vi "6733_write_waveform.vi"(8 "Error In":errorcluster, 9 "Control Task In":refnum<k21>, 10 "Waveform Task In":refnum<k21>, 11 "Inputs":T1 {"Waveform Parameters"."Degree (polynomial only)" min=1}) -> (0 "error out":errorcluster, 2 "counter task out":refnum<k21>, 3 "waveform task out":refnum<k21>)   [LabVIEW 2013]
uses:
  Control 1.ctl
  <vilib>/DAQmx/write.llb/DAQmx Write (Analog 1D DBL NChan 1Samp).vi
  <vilib>/DAQmx/write.llb/DAQmx Write (Analog 1D Wfm NChan NSamp).vi
  <vilib>/DAQmx/create/channels.llb/DAQmx Create Channel (AO-Voltage-Basic).vi
  <vilib>/DAQmx/miscellaneous.llb/DAQmx Fill In Error Info.vi
  <vilib>/Waveform/WDTOps.llb/WDT Append Waveforms DBL.vi
  <vilib>/DAQmx/configure/timing.llb/DAQmx Timing (Sample Clock).vi
  <vilib>/DAQmx/create/channels.llb/DAQmx Create Channel (CO-Pulse Generation-Frequency).vi
  <vilib>/DAQmx/configure/timing.llb/DAQmx Timing (Implicit).vi
  <vilib>/DAQmx/configure/trigger.llb/DAQmx Start Trigger (Digital Edge).vi
  <vilib>/Waveform/WDTOps.llb/WDT Scale Delta t DBL.vi
  <resource>/objmgr/daqmx.rc
panel:
  out "Total Time":dbl
  out "Sample Rate":dbl
  out "element":waveform(dbl)(graph)
  in  "index":i32
  out "Waveforms":waveform(dbl)[](array[waveform])
  out "Max Sample Rate":dbl=1000000.0
  out "# Inactive Channels":i32
  out "# Active Channels":i16
  out "Inactive Channels":tag[](array[tag])
  out "Active Channels":tag[](array[tag])
  out "Samples Written":dbl
  out "Voltage Maximum":dbl
  out "Voltage Minimum":dbl
  out "AO.PhysicalChans":tag[](array[tag])
  out "Active Device":tag
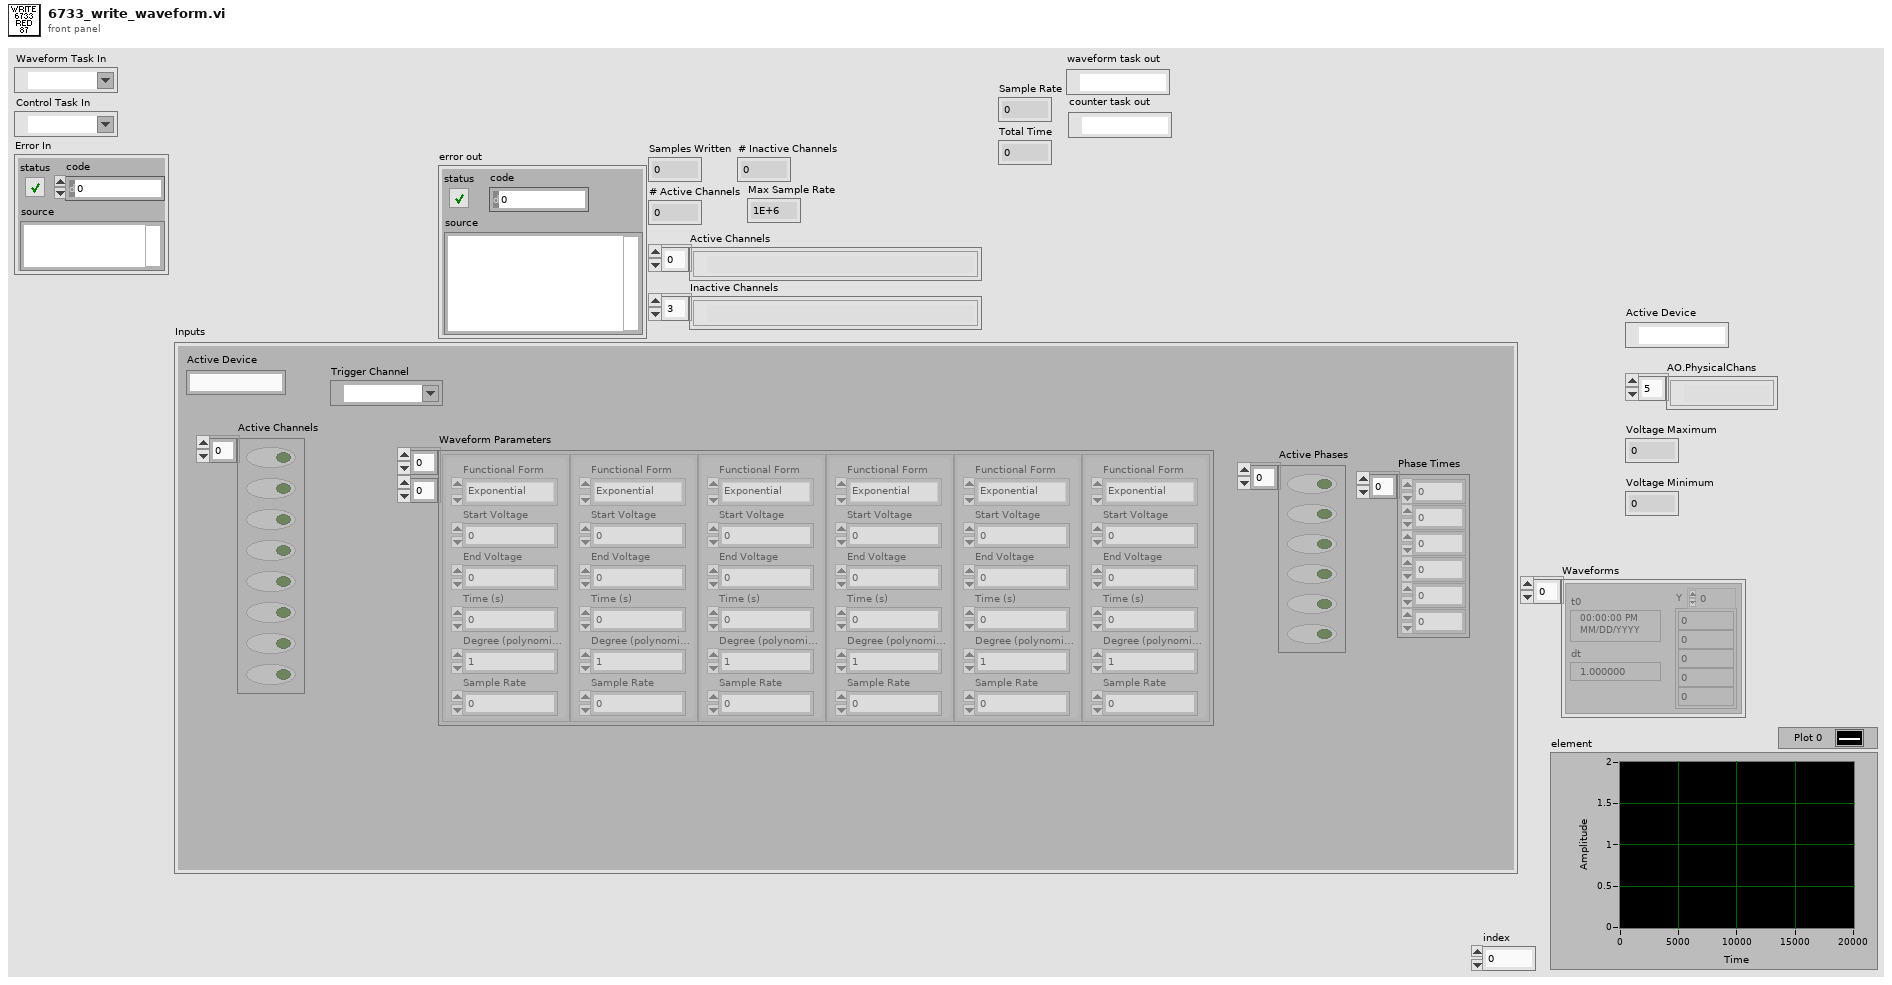
[diagram p1: front panel]
types:
  T1 = cluster{"Active Device":string, "Active Channels":bool[], "Waveform Parameters":cluster{"Functional Form":enum16{"Polynomial", "Exponential"}, "Start Voltage":dbl, "End Voltage":dbl, "Time (s)":dbl, "Degree (polynomial only)":i8, "Sample Rate":dbl}[][], "Active Phases":bool[], "Phase Times":dbl[], "Trigger Channel":tag}
  T2 = typedef "Control 1.ctl" = enum16{"Initialize", "Get Device Information", "Get Active/Inactive Channels", "Maximize Samples / Channel", "Write Waveforms", "Check for Problems", "Clear Old Tasks", "Write to cards"}
  T3 = cluster{"Functional Form":enum16{"Polynomial", "Exponential"}, "Start Voltage":dbl, "End Voltage":dbl, "Time (s)":dbl, "Degree (polynomial only)":i8, "Sample Rate":dbl}[][]
  T4 = cluster{"Functional Form":enum16{"Polynomial", "Exponential"}, "Start Voltage":dbl, "End Voltage":dbl, "Time (s)":dbl, "Degree (polynomial only)":i8, "Sample Rate":dbl}[]
  T5 = cluster{"Functional Form":enum16{"Polynomial", "Exponential"}, "Start Voltage":dbl, "End Voltage":dbl, "Time (s)":dbl, "Degree (polynomial only)":i8, "Sample Rate":dbl}
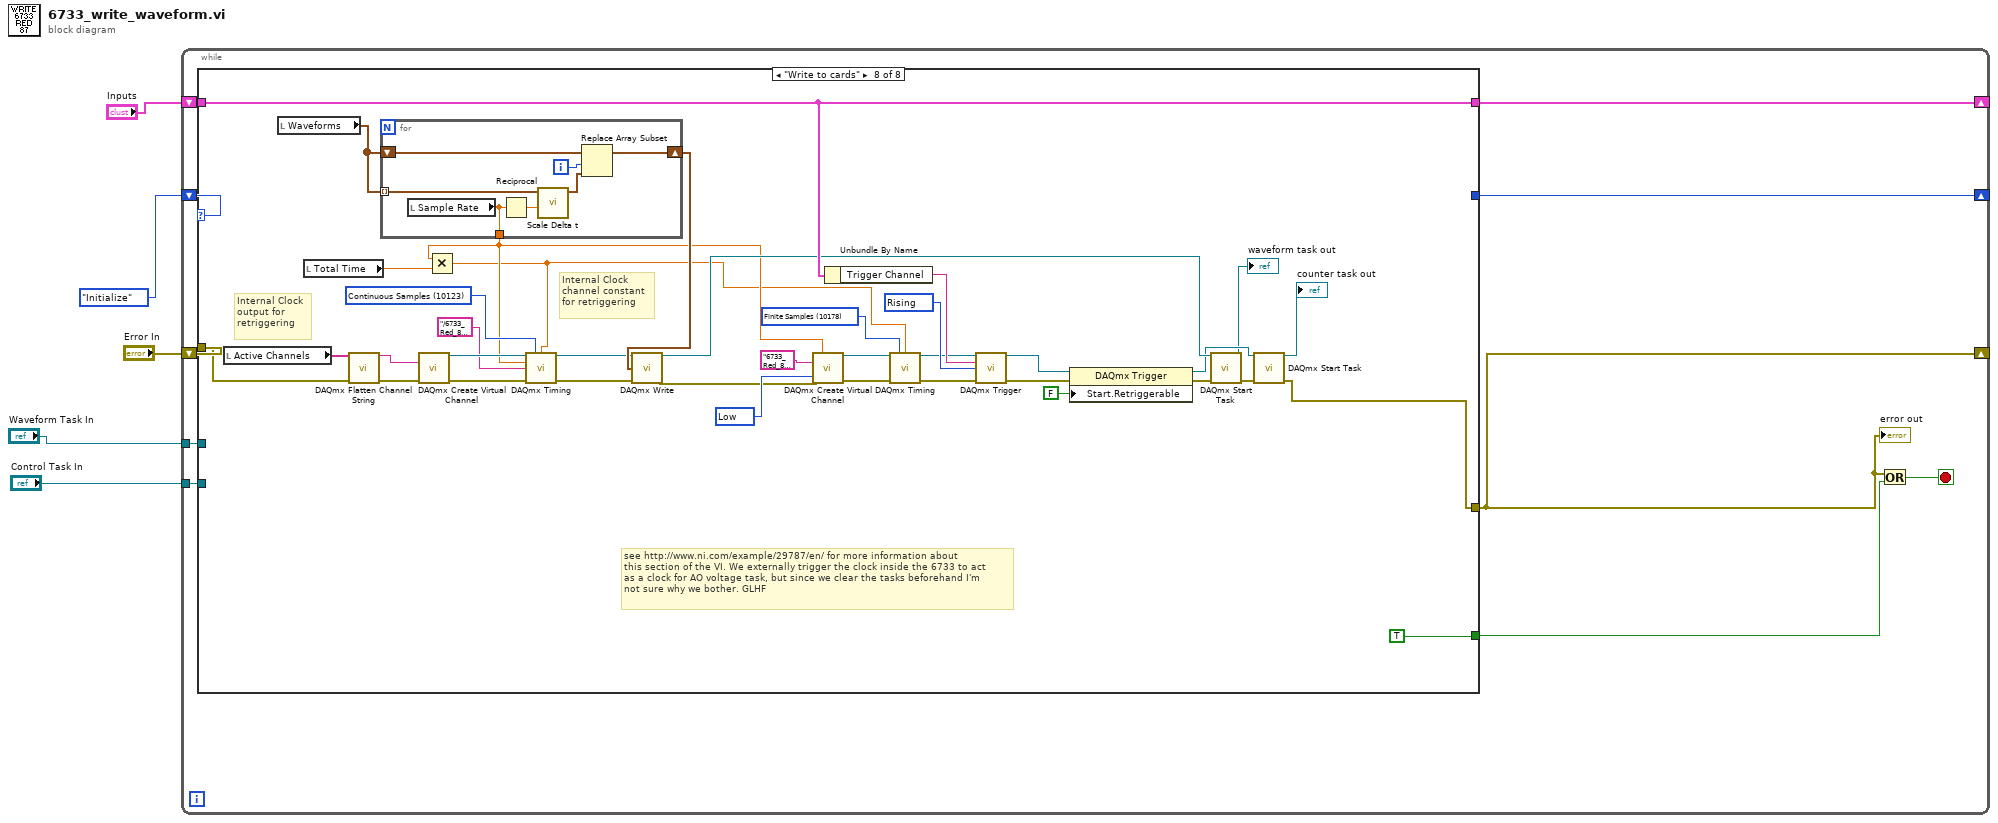
[diagram p0: block diagram]
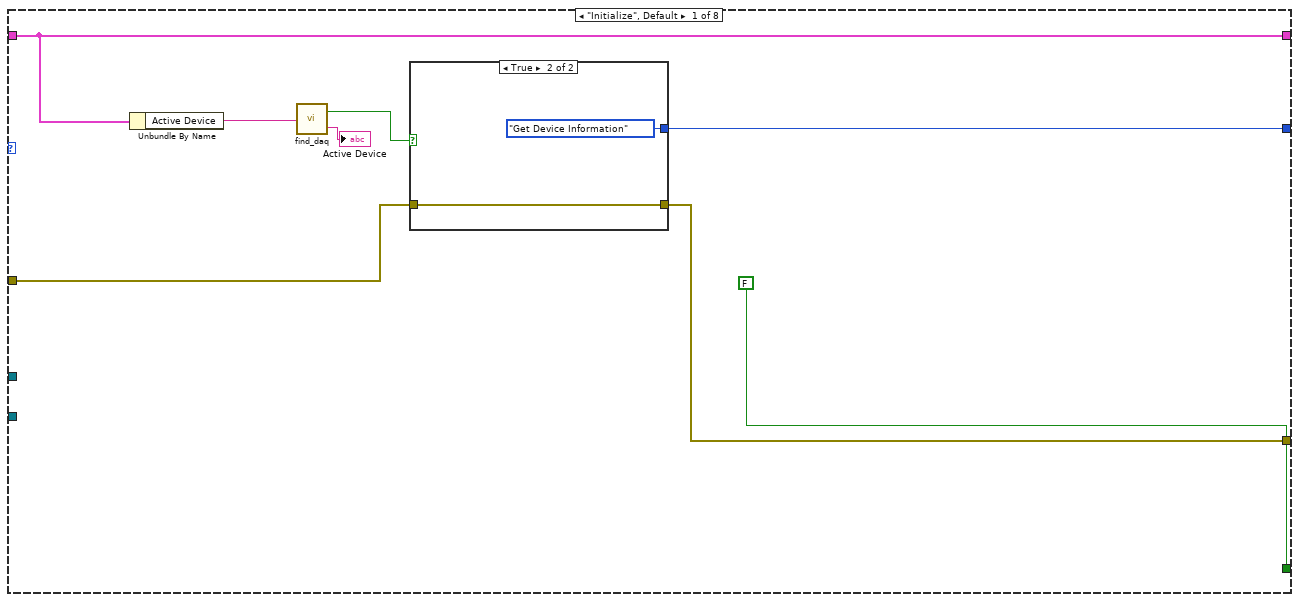
[diagram p2: hidden frame]
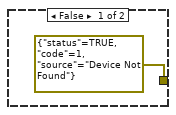
[diagram p3: hidden frame]
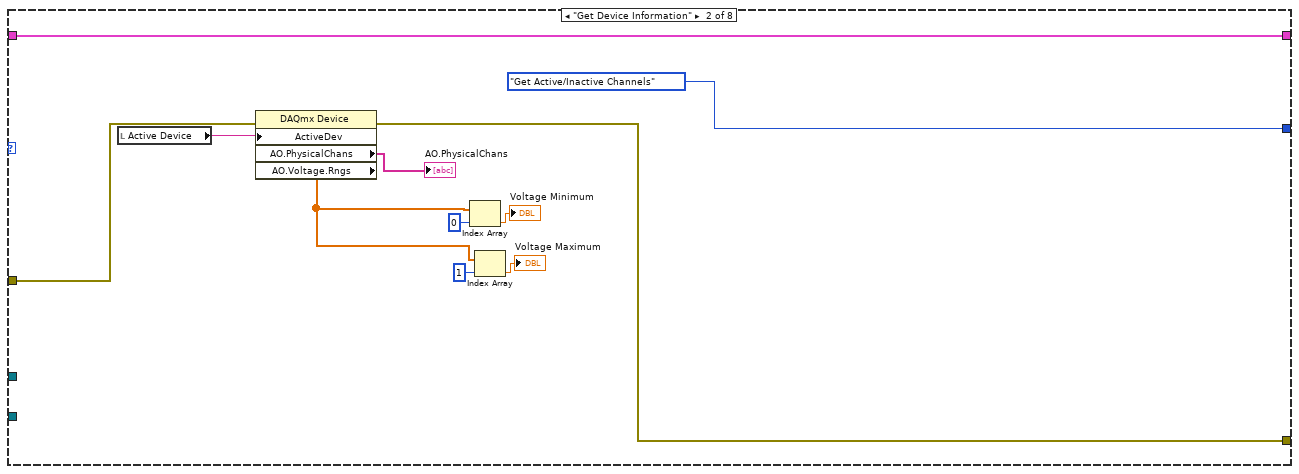
[diagram p4: hidden frame]
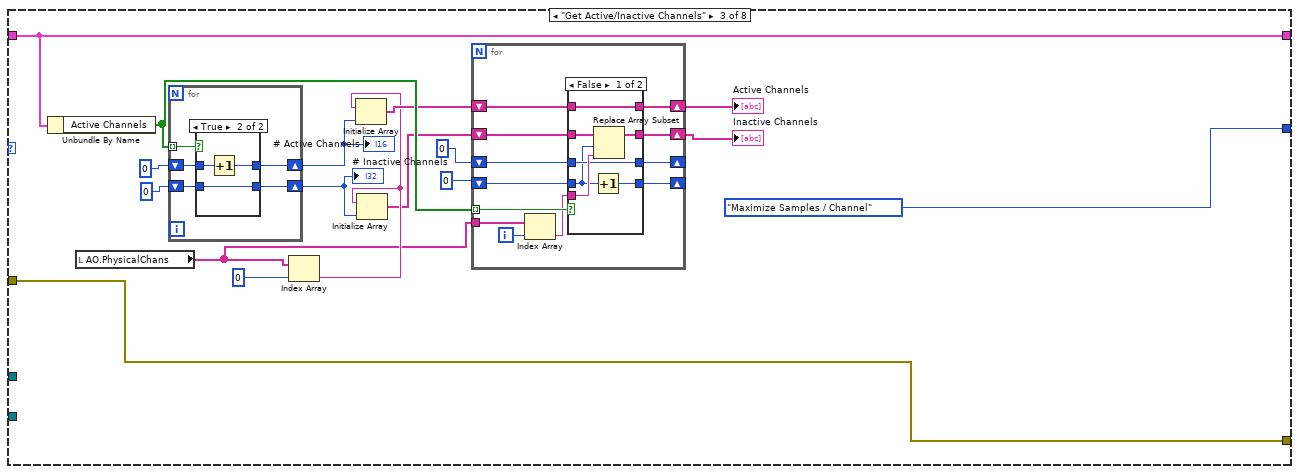
[diagram p5: hidden frame]
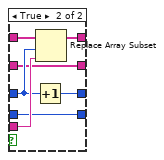
[diagram p6: hidden frame]
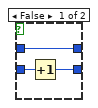
[diagram p7: hidden frame]
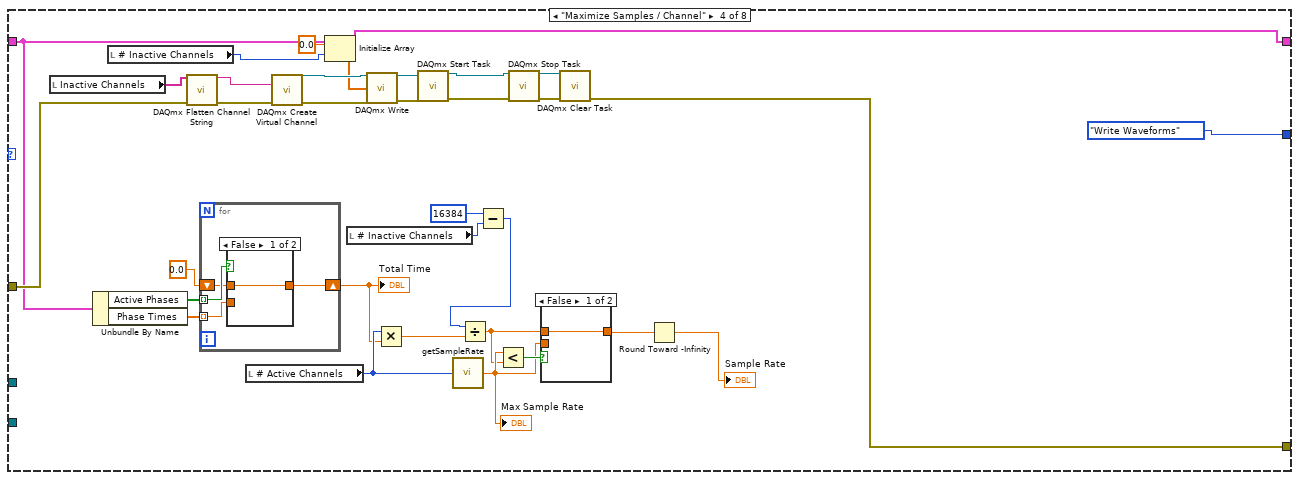
[diagram p8: hidden frame]
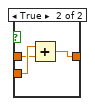
[diagram p10: hidden frame]
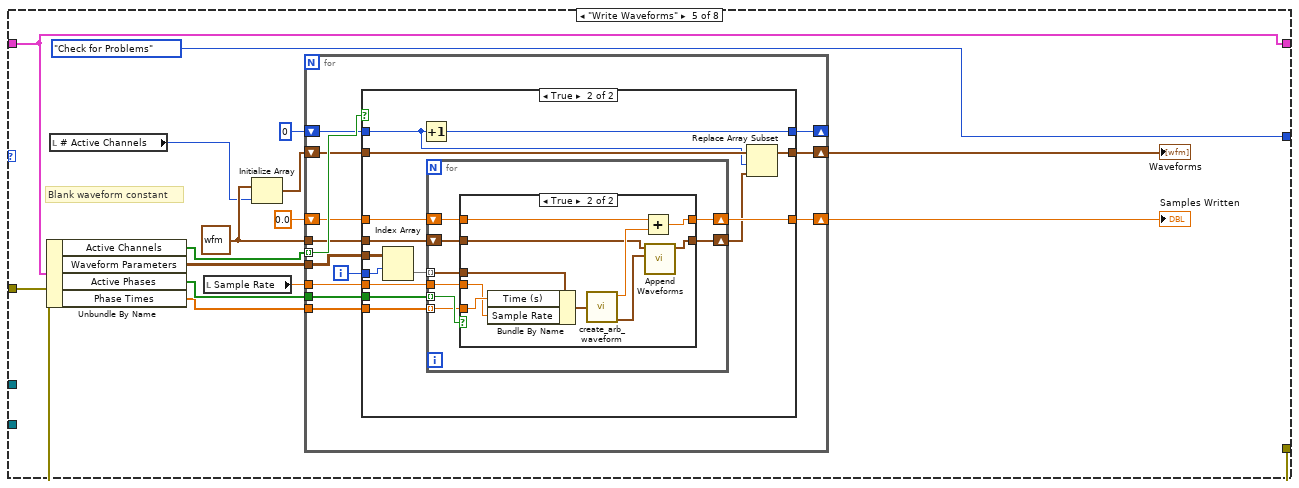
[diagram p11: hidden frame]
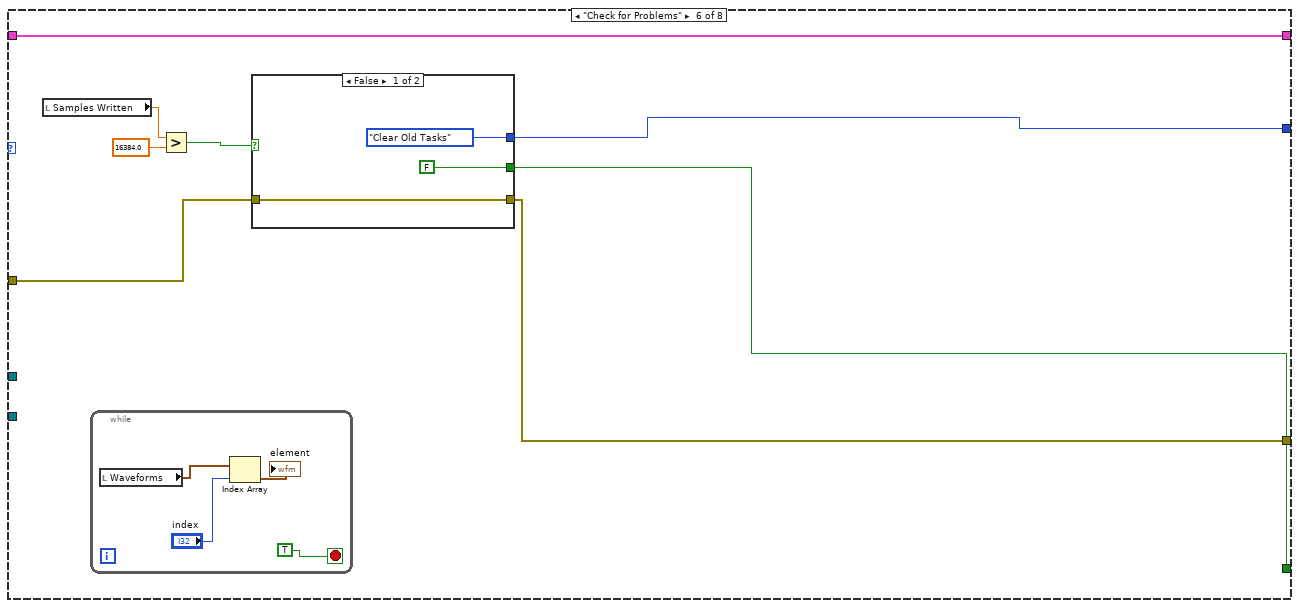
[diagram p14: hidden frame]
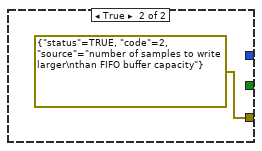
[diagram p15: hidden frame]
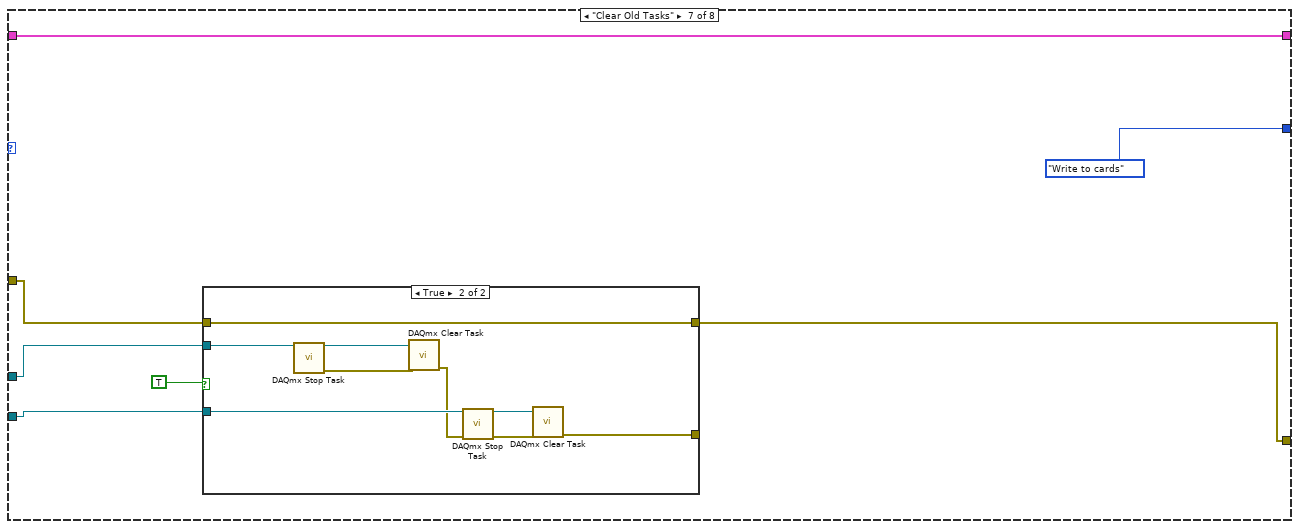
[diagram p16: hidden frame]
diagram:
  n1 = while {
    shift-right: [w11] -> _
    shift-left: "Error In" -> [w13]
    shift-right: [w12] -> _
    shift-left: Control_1."Initialize" -> [w15]
    shift-right: [w9] -> _
    shift-left: "Inputs" -> [w14]
    tunnel: "Control Task In" -> [w6]
    tunnel: "Waveform Task In" -> [w7]
    stop <- w10 stop-if-true
    n2 = case shown="\"Write to cards\"" w15 {
      tunnel: w14 -> [w17 w37 w41 w106 w144 w201 w215 w266]
      tunnel: [w20 w28 w52 w110 w147 w202 w218 w237] -> w11
      tunnel: w13 -> [w19 w36 w52 w121 w147 w203 w217 w265]
      tunnel: [w18 Control_1."Get Active/Inactive Channels" Control_1."Maximize Samples / Channel" Control_1."Write Waveforms" Control_1."Check for Problems" w200 Control_1."Write to cards" _] -> w12
      tunnel: [w17 w37 w41 w106 w144 w201 w215 w266] -> w9
      tunnel: [FALSE ("y") _ _ _ _ w199 _ TRUE ("y")] -> w8
      tunnel: w7 -> [_ _ _ _ _ _ w221 _]
      tunnel: w6 -> [_ _ _ _ _ _ w219 _]
      frame "Initialize", Default {
        n3 = Unbundle By Name(w17) -> ("Active Device"=w23:string)
        n4 = call "find_daq.vi"("Device Name"=w23) -> ("Device Present"=w21:bool, "DAQmx Device Name"=→"Active Device":tag)
        n5 = case shown="True" w21 {
          tunnel: [errorcluster {"status"=TRUE, "code"=1, "source"="Device Not Found"} ("error in (no error)") w26] -> w20
          tunnel: w19 -> [_ w26]
          tunnel: [_ Control_1."Get Device Information"] -> w18
          frame False {
          }
          frame True {
          }
        }
      }
      frame "Get Device Information" {
        n6 = local read "Active Device"() -> (w35:tag)
        n7 = property class="DAQmx Device"(error in=w36, "ActiveDev"=w35) -> (error out=w28:errorcluster, "AO.PhysicalChans"=→"AO.PhysicalChans":tag[], "AO.Voltage.Rngs"=w30:dbl[])  [unwired: 1 in, 1 out]
        n8 = Index Array(array=w30, index=0) -> (element=→"Voltage Minimum":dbl)
        n9 = Index Array(array=w30, index=1) -> (element=→"Voltage Maximum":dbl)
      }
      frame "Get Active/Inactive Channels" {
        n10 = Unbundle By Name(w41) -> ("Active Channels"=w51:bool[])
        n11 = local read "AO.PhysicalChans"() -> (w45:tag[])
        n12 = for {
          shift-right: [w85] -> w50
          shift-left: i16 0 -> [w84]
          shift-right: [w83] -> w49
          shift-left: 0 -> [w82]
          tunnel: w51 -> [w81] mode=indexing
          n13 = case shown="True" w81 {
            tunnel: [w86 w91] -> w85
            tunnel: w84 -> [w86 w90]
            tunnel: [w88 w89] -> w83
            tunnel: w82 -> [w87 w89]
            frame False {
              n14 = Increment(x=w87) -> (x+1=w88:i32)
            }
            frame True {
              n15 = Increment(x=w90) -> (x+1=w91:i16)
            }
          }
        }
        "# Active Channels" <- w50
        "# Inactive Channels" <- w49
        n16 = Index Array(array=w45, index=0) -> (element=w46:tag)
        n17 = Initialize Array(w46, w50) -> (w48:tag[])
        n18 = Initialize Array(w46, w49) -> (w44:tag[])
        n19 = for {
          tunnel: w51 -> [w66] mode=indexing
          shift-right: [w63] -> w40
          shift-left: w48 -> [w64]
          tunnel: w45 -> [w61]
          shift-right: [w59] -> w39
          shift-left: w44 -> [w60]
          shift-right: [w57] -> _
          shift-left: 0 ("index") -> [w58]
          shift-right: [w55] -> _
          shift-left: 0 ("index") -> [w56]
          i -> [w65]
          n20 = Index Array(array=w61, index=w65) -> (element=w62:tag)
          n21 = case shown="False" w66 {
            tunnel: w64 -> [w67 w80]
            tunnel: [w67 w79] -> w63
            tunnel: w62 -> [w73 w78]
            tunnel: w60 -> [w72 w74]
            tunnel: [w71 w74] -> w59
            tunnel: w58 -> [w70 w77]
            tunnel: [w70 w76] -> w57
            tunnel: w56 -> [w69 w75]
            tunnel: [w68 w75] -> w55
            frame False {
              n22 = Increment(x=w69) -> (x+1=w68:i32)
              n23 = Replace Array Subset(array=w72, new element=w73, index=w69) -> (w71:tag[])
            }
            frame True {
              n24 = Increment(x=w77) -> (x+1=w76:i32)
              n25 = Replace Array Subset(array=w80, new element=w78, index=w77) -> (w79:tag[])
            }
          }
        }
        "Active Channels" <- w40
        "Inactive Channels" <- w39
      }
      frame "Maximize Samples / Channel" {
        n26 = local read "Inactive Channels"() -> (w122:tag[])
        n27 = Unbundle By Name(w106) -> ("Active Phases"=w105:bool[], "Phase Times"=w104:dbl[])
        n28 = local read "# Inactive Channels"() -> (w115:i32)
        n29 = call <vilib>:"DAQmx Flatten Channel String.vi"("names in"=w122, "error in"=w121) -> ("names out"=w120:string, "error out"=w123:errorcluster)  [unwired: 12 in]
        n30 = for {
          tunnel: w105 -> [w129] mode=indexing
          tunnel: w104 -> [w128] mode=indexing
          shift-right: [w126] -> w97
          shift-left: 0.0 -> [w127]
          n31 = case shown="False" w129 {
            tunnel: w128 -> [_ w133]
            tunnel: w127 -> [w130 w132]
            tunnel: [w130 w131] -> w126
            frame False {
            }
            frame True {
              n32 = Add(x=w133, y=w132) -> (x+y=w131:dbl)
            }
          }
        }
        "Total Time" <- w97
        n33 = local read "# Active Channels"() -> (w98:i16)
        n34 = call-poly <vilib>:"DAQmx Create Virtual Channel.vi"("physical channels"=w120, "error in"=w123) -> ("task out"=w119:refnum<k21>, "error out"=w118:errorcluster)  [unwired: 12 in]
        n35 = Initialize Array(0.0 ("element"), w115) -> (w113:dbl[])
        n36 = local read "# Inactive Channels"() -> (w93:i32)
        n37 = call-poly <vilib>:"DAQmx Write.vi"("task/channels in"=w119, "data"=w113, "error in"=w118) -> ("task out"=w116:refnum<k21>, "error out"=w117:errorcluster)  [unwired: 10 in, 1 out]
        n38 = Multiply(x=w98, y=w97) -> (x*y=w99:dbl)
        n39 = call <vilib>:"DAQmx Start Task.vi"("task/channels in"=w116, "error in"=w117) -> ("task out"=w108:refnum<k21>, "error out"=w109:errorcluster)  [unwired: 12 in]
        n40 = call "getSampleRate.vi"("Number of active channels"=w98) -> ("Sample Rate"=w101:dbl)
        "Max Sample Rate" <- w101
        n41 = Subtract(x=16384, y=w93) -> (x-y=w92:i32)
        n42 = Divide(x=w92, y=w99) -> (x/y=w100:dbl)
        n43 = Less?(x=w101, y=w100) -> (x < y?=w102:bool)
        n44 = call <vilib>:"DAQmx Stop Task.vi"("task/channels in"=w108, "error in"=w109) -> ("task out"=w112:refnum<k21>, "error out"=w111:errorcluster)  [unwired: 12 in]
        n45 = case shown="False" w102 {
          tunnel: [w124 w125] -> w95
          tunnel: w101 -> [_ w125]
          tunnel: w100 -> [w124 _]
          frame False {
          }
          frame True {
          }
        }
        n46 = call <vilib>:"DAQmx Clear Task.vi"("task in"=w112, "error in"=w111) -> ("error out"=w110:errorcluster)  [unwired: 13 in]
        n47 = Round Toward -Infinity(1:w95) -> (0:→"Sample Rate":dbl)
      }
      frame "Write Waveforms" {
        w141 = waveform(dbl) {"t0"=timestamp(0 s since 1904-01-01), "dt"=1.0, "Y"=[]}
        # "Blank waveform constant"
        n48 = Unbundle By Name(w144) -> ("Active Channels"=w136:bool[], "Waveform Parameters"=w148:T3, "Active Phases"=w142:bool[], "Phase Times"=w137:dbl[])
        n49 = local read "# Active Channels"() -> (w134:i16)
        n50 = local read "Sample Rate"() -> (w135:dbl)
        n51 = Initialize Array(w141, w134) -> (w139:waveform(dbl)[])
        n52 = for {
          tunnel: w136 -> [w161] mode=indexing
          tunnel: w148 -> [w159]
          shift-right: [w158] -> w146
          shift-left: 0.0 -> [w157]
          tunnel: w142 -> [w156]
          tunnel: w141 -> [w155]
          shift-right: [w153] -> _
          shift-left: 0 -> [w154]
          shift-right: [w151] -> w138
          shift-left: w139 -> [w152]
          tunnel: w137 -> [w150]
          tunnel: w135 -> [w149]
          i -> [w160]
          n53 = case shown="True" w161 {
            tunnel: w160 -> [_ w178]
            tunnel: w159 -> [_ w177]
            tunnel: [w164 w176] -> w158
            tunnel: w157 -> [w164 w175]
            tunnel: w156 -> [_ w173]
            tunnel: w155 -> [_ w172]
            tunnel: w154 -> [w163 w169]
            tunnel: [w163 w171] -> w153
            tunnel: w152 -> [w162 w170]
            tunnel: [w162 w167] -> w151
            tunnel: w150 -> [_ w166]
            tunnel: w149 -> [_ w165]
            frame False {
            }
            frame True {
              n54 = Index Array(array=w177, index (row)=w178) -> (element=w174:T4)  [unwired: 1 in]
              n55 = Increment(x=w169) -> (x+1=w171:i32)
              n56 = for {
                shift-right: [w186] -> w176
                shift-left: w175 -> [w185]
                tunnel: w174 -> [w184] mode=indexing
                shift-right: [w182] -> w168
                shift-left: w172 -> [w183]
                tunnel: w173 -> [w181] mode=indexing
                tunnel: w166 -> [w180] mode=indexing
                tunnel: w165 -> [w179]
                n57 = case shown="True" w181 {
                  tunnel: [w188 w197] -> w186
                  tunnel: w185 -> [w188 w196]
                  tunnel: w184 -> [_ w192]
                  tunnel: w183 -> [w187 w194]
                  tunnel: [w187 w193] -> w182
                  tunnel: w180 -> [_ w191]
                  tunnel: w179 -> [_ w189]
                  frame False {
                  }
                  frame True {
                    n58 = Bundle By Name(cluster=w192, "Time (s)"=w191, "Sample Rate"=w189) -> (w190:T5)
                    n59 = call "create_arb_waveform.vi"("Waveform Parameters"=w190) -> ("Samples to Write"=w198:dbl, "output waveform"=w195:waveform(dbl))  [unwired: 2 out]
                    n60 = Add(x=w196, y=w198) -> (x+y=w197:dbl)
                    n61 = call-poly <vilib>:"Append Waveforms.vi"("waveform B"=w195, "waveform A"=w194) -> ("waveform out"=w193:waveform(dbl))  [unwired: 8 in, 1 out]
                  }
                }
              }
              n62 = Replace Array Subset(array=w170, new element=w168, index=w169) -> (w167:waveform(dbl)[])
            }
          }
        }
        "Samples Written" <- w146
        "Waveforms" <- w138
      }
      frame "Check for Problems" {
        n63 = local read "Samples Written"() -> (w206:dbl)
        n64 = while {
          stop <- TRUE stop-if-true
          n65 = local read "Waveforms"() -> (w210:waveform(dbl)[])
          n66 = Index Array(array=w210, index="index") -> (element=→"element":waveform(dbl))
        }
        n67 = Greater?(x=w206, y=16384.0) -> (0:w205:bool)
        n68 = case shown="False" w205 {
          tunnel: w203 -> [w213 _]
          tunnel: [w213 errorcluster {"status"=TRUE, "code"=2, "source"="number of samples to write larger\nthan FIFO buffer capacity"} ("error in (no error)")] -> w202
          tunnel: [Control_1."Clear Old Tasks" _] -> w200
          tunnel: [FALSE ("y") _] -> w199
          frame False {
          }
          frame True {
          }
        }
      }
      frame "Clear Old Tasks" {
        n69 = case shown="True" TRUE {
          tunnel: w221 -> [_ w231]
          tunnel: w219 -> [_ w229]
          tunnel: [w222 w227] -> w218
          tunnel: w217 -> [w222 w227]
          tunnel: [_ w223] -> _
          frame False {
          }
          frame True {
            n70 = call <vilib>:"DAQmx Stop Task.vi"("task/channels in"=w231) -> ("task out"=w230:refnum<k21>, "error out"=w226:errorcluster)  [unwired: 13 in]
            n71 = call <vilib>:"DAQmx Clear Task.vi"("task in"=w230, "error in"=w226) -> ("error out"=w225:errorcluster)  [unwired: 13 in]
            n72 = call <vilib>:"DAQmx Stop Task.vi"("task/channels in"=w229, "error in"=w225) -> ("task out"=w228:refnum<k21>, "error out"=w224:errorcluster)  [unwired: 12 in]
            n73 = call <vilib>:"DAQmx Clear Task.vi"("task in"=w228, "error in"=w224) -> ("error out"=w223:errorcluster)  [unwired: 13 in]
          }
        }
      }
      frame "Write to cards" {
        w250 = 10280 items=["Rising"=10280, "Falling"=10171] ("edge")
        w257 = 10123 items=["Finite Samples"=10178, "Continuous Samples"=10123, "Hardware Timed Single Point"=12522] ("sample mode")
        w259 = 10178 items=["Finite Samples"=10178, "Continuous Samples"=10123, "Hardware Timed Single Point"=12522] ("sample mode")
        w262 = 10214 items=["High"=10192, "Low"=10214] ("idle state")
        # "see http://www.ni.com/example/29787/en/ for more information about\nthis section of the VI. We externally trigger the clock inside the 6733 to act\nas a clock for AO voltage task, but since we clear the tasks beforehand I'm\nnot sure why we bother. GLHF"
        # "Internal Clock\noutput for\nretriggering"
        # "Internal Clock\nchannel constant\nfor retriggering"
        n74 = local read "Active Channels"() -> (w264:tag[])
        n75 = local read "Waveforms"() -> (w267:waveform(dbl)[])
        n76 = local read "Total Time"() -> (w258:dbl)
        n77 = call <vilib>:"DAQmx Flatten Channel String.vi"("names in"=w264, "error in"=w265) -> ("names out"=w263:string, "error out"=w234:errorcluster)  [unwired: 12 in]
        n78 = for {
          tunnel: w267 -> [w275] mode=indexing
          shift-right: [w269] -> w253
          shift-left: w267 -> [w271]
          tunnel: [w270] -> w240
          i -> [w273]
          n79 = local read "Sample Rate"() -> (w270:dbl)
          n80 = Reciprocal(x=w270) -> (1/x=w274:dbl)
          n81 = call-poly <vilib>:"Scale Delta t.vi"("scale factor"=w274, "waveform in"=w275) -> ("waveform out"=w272:waveform(dbl))  [unwired: 8 in, 1 out]
          n82 = Replace Array Subset(array=w271, new element=w272, index=w273) -> (w269:waveform(dbl)[])
        }
        n83 = call-poly <vilib>:"DAQmx Create Virtual Channel.vi"("physical channels"=w263, "error in"=w234) -> ("task out"=w256:refnum<k21>, "error out"=w255:errorcluster)  [unwired: 12 in]
        n84 = Multiply(x=w240, y=w258) -> (x*y=w232:dbl)
        n85 = call-poly <vilib>:"DAQmx Timing.vi"("task/channels in"=w256, "sample mode"=w257, "samples per channel"=w232, "rate"=w240, "source"=tag "/6733_Red_87/Ctr0InternalOutput", "error in"=w255) -> ("task out"=w252:refnum<k21>, "error out"=w254:errorcluster)  [unwired: 8 in]
        n86 = call-poly <vilib>:"DAQmx Write.vi"("task/channels in"=w252, "data"=w253, "error in"=w254) -> ("task out"=w244:refnum<k21>, "error out"=w233:errorcluster)  [unwired: 10 in, 1 out]
        n87 = call-poly <vilib>:"DAQmx Create Virtual Channel.vi"("frequency"=w240, "counter"=tag "6733_Red_87/ctr0", "error in"=w233, "idle state"=w262) -> ("task out"=w261:refnum<k21>, "error out"=w260:errorcluster)  [unwired: 10 in]
        n88 = Unbundle By Name(w266) -> ("Trigger Channel"=w249:tag)
        n89 = call-poly <vilib>:"DAQmx Timing.vi"("task/channels in"=w261, "sample mode"=w259, "samples per channel"=w232, "error in"=w260) -> ("task out"=w248:refnum<k21>, "error out"=w251:errorcluster)  [unwired: 10 in]
        n90 = call-poly <vilib>:"DAQmx Trigger.vi"("task/channels in"=w248, "source"=w249, "edge"=w250, "error in"=w251) -> ("task out"=w246:refnum<k21>, "error out"=w247:errorcluster)  [unwired: 10 in]
        n91 = property class="DAQmx Trigger"(reference=w246, error in=w247, "Start.Retriggerable"=FALSE) -> (reference out=w241:refnum<k21>, error out=w243:errorcluster)
        n92 = call <vilib>:"DAQmx Start Task.vi"("task/channels in"=w244, "error in"=w243) -> ("task out"=→"waveform task out":refnum<k21>, "error out"=w242:errorcluster)  [unwired: 12 in]
        n93 = call <vilib>:"DAQmx Start Task.vi"("task/channels in"=w241, "error in"=w242) -> ("task out"=→"counter task out":refnum<k21>, "error out"=w237:errorcluster)  [unwired: 12 in]
      }
    }
    "error out" <- w11
    n94 = Or(x=w11, y=w8) -> (x .or. y?=w10:bool)
  }
